vi "Read Relay.vi"() -> (1 "unsigned 8bit integer":u8, 2 "Boolean array":bool[](array[boolean]))   [LabVIEW 2019, in "Relay-Box.lvclass"]
uses:
  <userlib>/LevyLab/Relay Box/Relay-Box.lvclass
  <userlib>/LevyLab/Relay Box/Relay-Box.lvclass/Relay-Box.ctl
  <userlib>/LevyLab/Relay Box/D2XX_Functions/D2XX_Functions.lvlib
panel:
  out "error out":errorcluster
  in  "error in (no error)":errorcluster
  out "FT_Status out":u32(ring) items=["FT_OK", "FT_INVALID_HANDLE", "FT_DEVICE_NOT_FOUND", "FT_DEVICE_NOT_OPENED", "FT_IO_ERROR", "FT_INSUFFICIENT_RESOURCES", "FT_INVALID_PARAMETER", "FT_INVALID_BAUD_RATE", "FT_DEVICE_NOT_OPENED_FOR_ERASE", "FT_DEVICE_NOT_OPENED_FOR_WRITE", "FT_FAILED_TO_WRITE_DEVICE", "FT_EEPROM_READ_FAILED", "FT_EEPROM_WRITE_FAILED", "FT_EEPROM_ERASE_FAILED", "FT_EEPROM_NOT_PRESENT", "FT_EEPROM_NOT_PROGRAMMED", "FT_INVALID_ARGS", "FT_NOT_SUPPORTED", "FT_OTHER_ERROR"]
  # "Discharge tip"
  # "0 ohm"
  # "100k ohm"
  # "10M ohm"
  # "1Gohm"
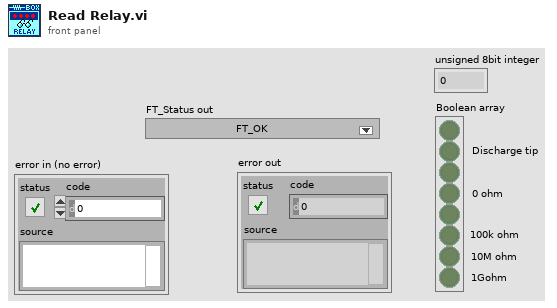
[diagram p1: front panel]
types:
  T1 = cluster{"Vendor ID":u16, "Product ID":u16, "Manufacturer":string, "Manufacturer ID":string, "Description":string, "Serial Number":string, "Max Power (mA)":u16, "PnP":u16, "Self Powered":u16, "Remote Wake-Up":u16, "Use Ext Osc":u8, "High Drive IOs":u8, "Endpoint Size":u8, "Pull Down Enable":u8, "Serial Number Enable":u8, "Invert TXD":u8, "Invert RXD":u8, "Invert RTS":u8, "Invert CTS":u8, "Invert DTR":u8, "Invert DSR":u8, "Invert DCD":u8, "Invert RI":u8, "CBus0":u8, "CBus1":u8, "CBus2":u8, "CBus3":u8, "CBus4":u8, "Is D2XX":u8}
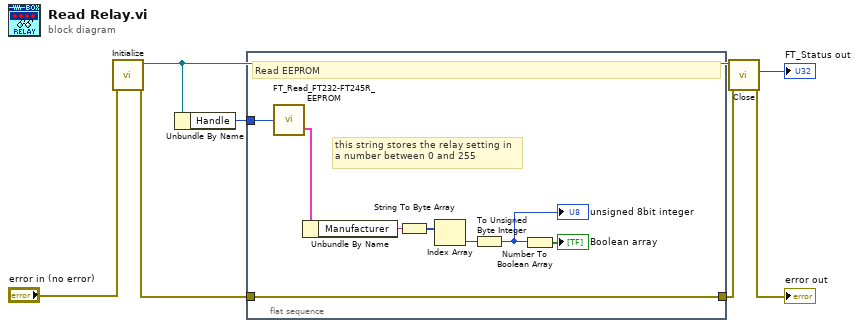
[diagram p0: block diagram]
diagram:
  n1 = call <userlib>:"Initialize.vi"("error in (no error)"="error in (no error)") -> ("error out"=w4:errorcluster, "Relay-Box out"=w6:refnum<class "Relay-Box.lvclass">)  [unwired: 9 in]
  n2 = Unbundle By Name(w6) -> ("Handle"=w7:u32)
  n3 = flat-sequence {
    tunnel: [w10] -> w2
    tunnel: w7 -> [w11]
    tunnel: w4 -> [w10]
    frame #0 {
      # "this string stores the relay setting in\na number between 0 and 255"
      # "Read EEPROM"
      n4 = call <userlib>:"FT_Read_FT232-FT245R_EEPROM.vi"("Handle"=w11) -> ("FT232-FT245R EEPROM Contents"=w9:T1)  [unwired: 1 out]
      n5 = Unbundle By Name(w9) -> ("Manufacturer"=w15:string)
      n6 = String To Byte Array(string=w15) -> (unsigned byte array=w14:u8[])
      n7 = Index Array(array=w14) -> (element=w8:u8)  [unwired: 1 in]
      n8 = To Unsigned Byte Integer(number=w8) -> (unsigned 8bit integer=w13:u8)
      "unsigned 8bit integer" <- w13
      n9 = Number To Boolean Array(number=w13) -> (Boolean array=→"Boolean array":bool[])
    }
  }
  n10 = call <userlib>:"Close.vi"("error in (no error)"=w2, "Relay-Box in"=w6) -> ("error out"=→"error out":errorcluster, "FT_Status"=→"FT_Status out":u32)  [unwired: 7 in, 1 out]
